vi "ILC Errors.vi"(8 "error in (no error)":errorcluster, 11 "[error code] (0)":i32 format="%0.0f") -> (0 "error out":errorcluster)   [LabVIEW 2014]
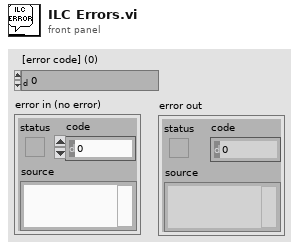
[diagram p1: front panel]
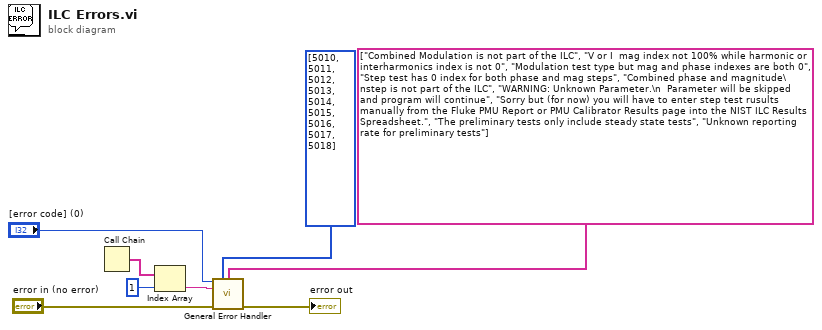
[diagram p0: block diagram]
diagram:
  n1 = Call Chain() -> (call chain=w3:string[])
  n2 = Index Array(array=w3, index=1) -> (element=w1:string)
  n3 = call <vilib>:"General Error Handler.vi"("[error code] (0)"="[error code] (0)", "[user-defined codes]"=i32[] [5010, 5011, 5012, 5013, 5014, 5015, 5016, 5017, 5018], "[user-defined descriptions]"=string[] ["Combined Modulation is not part of the ILC", "V or I  mag index not 100% while harmonic or interharmonics index is not 0", "Modulation test type but mag and phase indexes are both 0", "Step test has 0 index for both phase and mag steps", "Combined phase and magnitude\nstep is not part of the ILC", "WARNING: Unknown Parameter.\n  Parameter will be skipped and program will continue", "Sorry but (for now) you will have to enter step test rusults manually from the Fluke PMU Report or PMU Calibrator Results page into the NIST ILC Results Spreadsheet.", "The preliminary tests only include steady state tests", "Unknown reporting rate for preliminary tests"], "[error source] (\" \")"=w1, "error in (no error)"="error in (no error)") -> ("error out"=→"error out":errorcluster)  [unwired: 6 in, 4 out]
